vi "Gif.ColorTable.vi"(0 "data":string, 5 "flag":u8, 7 "Size of Color Table":u8, 9 "offset":i32, 11 "error in (no error)":errorcluster) -> (4 "data out":string, 6 "color table":u32[](array[numeric]), 10 "offset out":i32, 15 "error out":errorcluster)   [LabVIEW 2019]
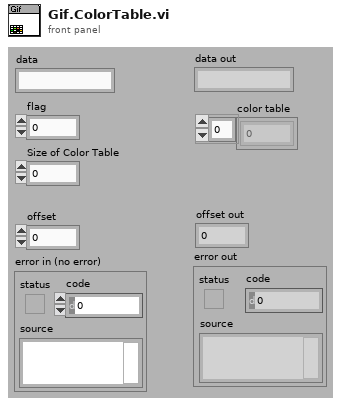
[diagram p1: front panel]
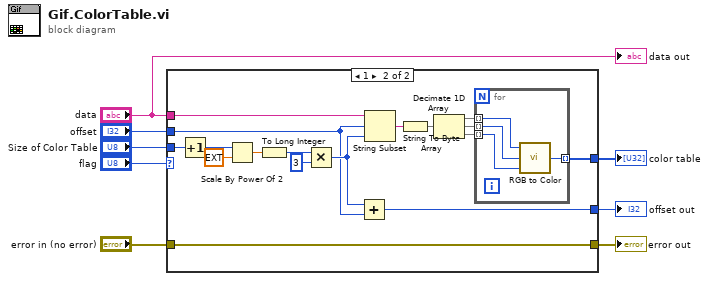
[diagram p0: block diagram]
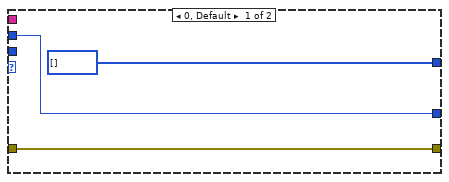
[diagram p2: hidden frame]
diagram:
  n1 = case shown="1" "flag" {
    tunnel: "Size of Color Table" -> [_ w28]
    tunnel: "offset" -> [w11 w20]
    tunnel: "data" -> [_ w22]
    tunnel: [u32[] [] w14] -> w4
    tunnel: [w11 w13] -> w3
    tunnel: "error in (no error)" -> [w9 w12]
    tunnel: [w9 w12] -> w1
    frame 0, Default {
    }
    frame 1 {
      n2 = Increment(x=w28) -> (x+1=w27:u8)
      n3 = Scale By Power Of 2(n=w27, x=ext 1.0) -> (x*2^n=w25:ext)
      n4 = To Long Integer(number=w25) -> (32bit integer=w24:i32)
      n5 = Multiply(x=w24, y=3) -> (x*y=w21:i32)
      n6 = Add(x=w21, y=w20) -> (x+y=w13:i32)
      n7 = String Subset(string=w22, offset (0)=w20, length (rest)=w21) -> (substring=w19:string)
      n8 = String To Byte Array(string=w19) -> (unsigned byte array=w18:u8[])
      n9 = Decimate 1D Array(w18) -> (w17:u8[], w16:u8[], w15:u8[])
      n10 = for {
        tunnel: w17 -> [w30] mode=indexing
        tunnel: w16 -> [w32] mode=indexing
        tunnel: w15 -> [w29] mode=indexing
        tunnel: [w31] -> w14 mode=indexing
        n11 = call <vilib>:"RGB to Color.vi"("B"=w29, "G"=w32, "R"=w30) -> ("Color"=w31:u32)
      }
    }
  }
  "error out" <- w1
  "color table" <- w4
  "offset out" <- w3
  "data out" <- "data"
